vi "getIPAddress.vi"(1 "Computer Name":string) -> (0 "IP Address":string)   [LabVIEW 2018, in "TcpServer.lvclass"]
doc: "Get IP address from configServer.vi"
uses:
  TcpServer.lvclass
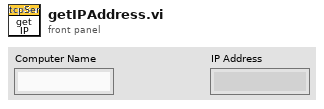
[diagram p1: front panel]
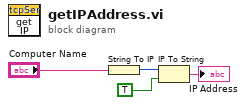
[diagram p0: block diagram]
diagram:
  n1 = String To IP(1:"Computer Name") -> (0:w4:u32)
  n2 = IP To String(1:TRUE ("dot notation? (F)"), 2:w4) -> (0:→"IP Address":string)
